vi "CVT Bool IndexWrite.vi"(3 "error in (no error)":errorcluster, 4 "Value":bool, 5 "Tag Index":i32) -> (0 "error out":errorcluster)   [LabVIEW 2020, in "Current Value Table(Rebuild).lvlib"]
uses:
  Current Value Table(Rebuild).lvlib
  DataTypes/Boolean_Write Index.vi
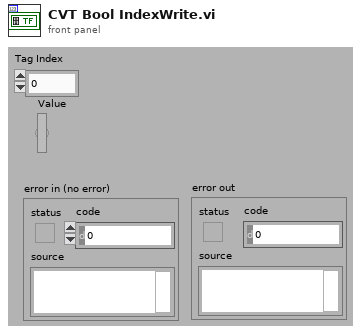
[diagram p1: front panel]
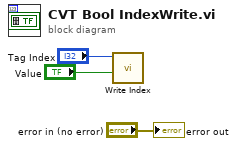
[diagram p0: block diagram]
diagram:
  n1 = call-poly "Write Index.vi"("Value"="Value", "Index"="Tag Index") -> ()  [unwired: 10 in]
  "error out" <- "error in (no error)"
